vi "GUI_channel.vi"(8 "error in (no error)":errorcluster, 11 "Thorlabs_OSA_64 in":refnum<class "OSA.lvclass">) -> (0 "error out":errorcluster, 3 "Thorlabs_OSA_64 out":refnum<class "OSA.lvclass">)   [LabVIEW 2010, in "OSA.lvclass"]
uses:
  OSA.lvclass
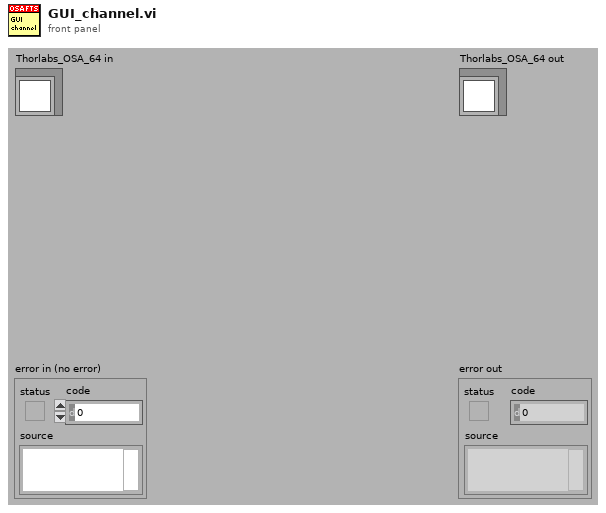
[diagram p1: front panel]
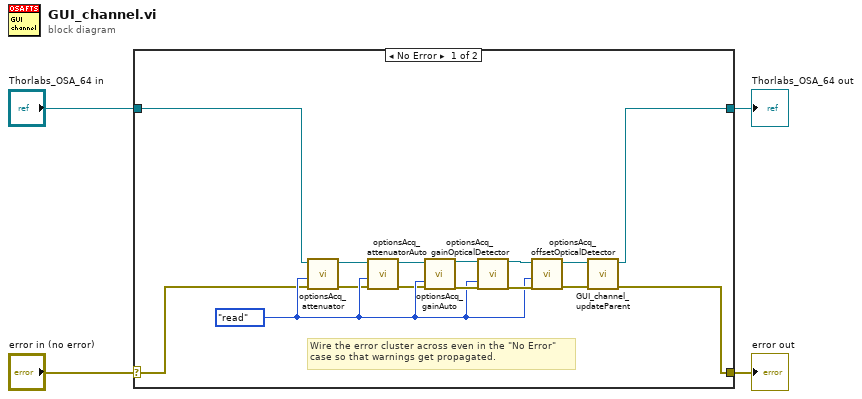
[diagram p0: block diagram]
diagram:
  n1 = case shown="No Error" "error in (no error)" {
    selector: "error in (no error)" -> [w12 w21]
    tunnel: [w5 w21] -> w3
    tunnel: [w6 w20] -> w1
    tunnel: "Thorlabs_OSA_64 in" -> [w7 w20]
    frame No Error {
      w13 = enum16{"read", "write"}."read" ("readWrite")
      # "Wire the error cluster across even in the \"No Error\"\ncase so that warnings get propagated."
      n2 = call-dynamic "optionsAcq_attenuator.vi"("error in (no error)"=w12, "readWrite"=w13, "Thorlabs_OSA_64 in"=w7) -> ("error out"=w11:errorcluster, "Thorlabs_OSA_64 out"=w9:refnum<class "OSA.lvclass">)  [unwired: 4 in, 3 out]
      n3 = call-dynamic "optionsAcq_attenuatorAuto.vi"("error in (no error)"=w11, "readWrite"=w13, "Thorlabs_OSA_64 in"=w9) -> ("error out"=w10:errorcluster, "Thorlabs_OSA_64 out"=w8:refnum<class "OSA.lvclass">)  [unwired: 5 in, 2 out]
      n4 = call-dynamic "optionsAcq_gainAuto.vi"("reference"=w8, "readWrite"=w13, "error in (no error)"=w10) -> ("duplicate reference"=w14:refnum<class "OSA.lvclass">, "error out"=w15:errorcluster)  [unwired: 13 in, 2 out]
      n5 = call-dynamic "optionsAcq_gainOpticalDetector.vi"("reference"=w14, "readWrite"=w13, "error in (no error)"=w15) -> ("duplicate reference"=w16:refnum<class "OSA.lvclass">, "error out"=w19:errorcluster)  [unwired: 12 in, 3 out]
      n6 = call-dynamic "optionsAcq_offsetOpticalDetector.vi"("error in (no error)"=w19, "readWrite"=w13, "Thorlabs_OSA_64 in"=w16) -> ("error out"=w18:errorcluster, "Thorlabs_OSA_64 out"=w17:refnum<class "OSA.lvclass">)  [unwired: 5 in, 2 out]
      n7 = call-dynamic "GUI_channel_updateParent.vi"("error in (no error)"=w18, "Thorlabs_OSA_64 in"=w17) -> ("error out"=w5:errorcluster, "Thorlabs_OSA_64 out"=w6:refnum<class "OSA.lvclass">)  [unwired: 8 in]
    }
    frame Error {
    }
  }
  "error out" <- w3
  "Thorlabs_OSA_64 out" <- w1
